vi "WriteReadSPIforAD5781-TEST.vi"() -> ()   [LabVIEW 2014]
uses:
  Host API/Controls/FPGA Reference.ctl
  <vilib>/rvi/interface/nirviOpenFPGA/nirviOpenFPGA.xnode
  FPGA Bitfiles/SPIExample_FPGATarget3_FPGASPIFPGATopLe_SKx8rjJlgp0.lvbitx
  FPGA/FPGA SPI_FPGA Top Level.vi
  <vilib>/rvi/interface/nirviMethod/nirviMethod.xnode
  Host API/Controls/SPI Configuration Cluster.ctl
  <vilib>/rvi/interface/nirviCloseFPGA/nirviCloseFPGA.xnode
  <vilib>/rvi/errors/niLvFpgaMergeErrorWithErrorCode.vi
panel:
  in  "Set Volt":bool
  in  "millisecond multiple":u32
  in  "Set Volt":u32 max=262143 format="%018b"
  in  "stop":bool
  out "Read Data":u8[](array[numeric]) format="%08b"
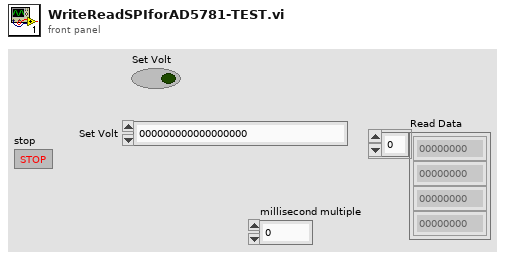
[diagram p1: front panel]
types:
  T1 = typedef "SPI Configuration Cluster.ctl" = cluster{"CS":u8, "Clock Rate (Hz)":dbl, "Clock Mode":u8, "CS Active State":bool}
  T2 = cluster{"Port":i8, "Configuration Cluster":T1, "Hardware Pins":cluster{"RESET":bool, "LDAC":bool, "CLR":bool}, "Total Bits":u16}
  T3 = typedef "FPGA Reference.ctl" = refnum<k20>
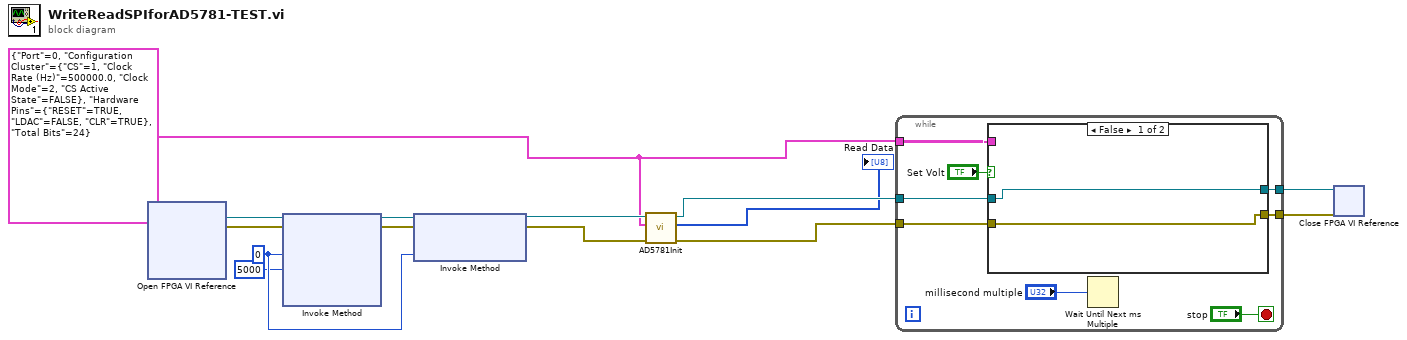
[diagram p0: block diagram]
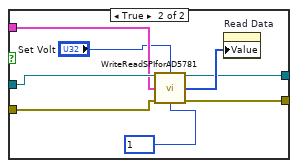
[diagram p2: hidden frame]
diagram:
  w5 = T2 {"Port"=0, "Configuration Cluster"={"CS"=1, "Clock Rate (Hz)"=500000.0, "Clock Mode"=2, "CS Active State"=FALSE}, "Hardware Pins"={"RESET"=TRUE, "LDAC"=FALSE, "CLR"=TRUE}, "Total Bits"=24} ("SPI - AD5781 Setup")
  w14 = 0 ("IRQ Number(s)")
  n1 = xnode "Open FPGA VI Reference"() -> ("FPGA VI Reference Out"=w9:T3, "error out"=w10:errorcluster)  [unwired: 2 in]
  n2 = xnode "Invoke Method"("FPGA VI Reference In"=w9, "error in"=w10, "IRQ Number(s)"=w14, "Timeout (ms)"=5000) -> ("FPGA VI Reference Out"=w11:T3, "error out"=w12:errorcluster)  [unwired: 2 out]
  n3 = xnode "Invoke Method"("FPGA VI Reference In"=w11, "error in"=w12, "IRQ Number(s)"=w14) -> ("FPGA VI Reference Out"=w6:T3, "error out"=w4:errorcluster)
  n4 = call "AD5781Init.vi"("error in"=w4, "SPI - AD5781 Setup"=w5, "FPGA Interface"=w6) -> ("error out"=w3:errorcluster, "Read Data"=→"Read Data":u8[], "FPGA Interface 2"=w2:T3)  [unwired: 6 in]
  n5 = while {
    tunnel: w3 -> [w20]
    tunnel: w2 -> [w21]
    tunnel: w5 -> [w19]
    tunnel: [w18] -> w7
    tunnel: [w17] -> w8
    stop <- "stop" stop-if-true
    n6 = case shown="False" "Set Volt" {
      tunnel: w21 -> [w24 w32]
      tunnel: w20 -> [w23 w31]
      tunnel: w19 -> [_ w30]
      tunnel: [w23 w27] -> w18
      tunnel: [w24 w26] -> w17
      frame False {
      }
      frame True {
        n7 = call "WriteReadSPIforAD5781.vi"("FPGA VI Reference Out 2"=w32, "DAC 18Bit Data"="Set Volt", "SPI - AD5781 Setup"=w30, "error in"=w31, "register prefix"=u8 1) -> ("FPGA VI Reference Out"=w26:T3, "Read Data"=w28:u8[], "error out"=w27:errorcluster)  [unwired: 8 in]
        n8 = property on="Read Data" class="Arr (strict)"("Value"=w28) -> ()  [unwired: 2 in, 2 out]
      }
    }
    n9 = Wait Until Next ms Multiple(millisecond multiple="millisecond multiple") -> ()  [unwired: 1 out]
  }
  n10 = xnode "Close FPGA VI Reference"("FPGA VI Reference In"=w8, "error in"=w7) -> ()  [unwired: 1 out]
